vi "Obtaining Known Object Reference.vi"() -> ()   [LabVIEW 2023]
doc: "This scripting VI locates the Edit me control in the target VI and changes the Representation of the control. Because the Edit me control has a unique label, this VI can easily access it with the Open VI Object Reference function.\n\nThe Detailed Help explains how this example illustrates a general procedure for obtaining a reference in a known target VI."
uses:
  <vilib>/numeric/LVNumericRepresentation.ctl
panel:
  in  "Edit me":string="Edit me"
  # "Select Help>>Show Context Help and move the cursor over the VI icon to display help for this VI.\n\nBefore you start: Open the Detailed Help for this example to display the Obtaining References to Objects in a Known Target VI Using VI Scripting topic in the  LabVIEW Help. That topic provides additional details about how this example illustrates the general procedure for obtaining a reference to an object in a known target VI using VI Scripting.\n\nThis scripting VI locates the Edit me control in the target VI and changes the numeric representation of that control to I32. Because the Edit me control has a unique label, this VI can easily access it with the Open VI Object Reference function.\n\nOpen the target VI to observe the effects of this scripting VI. The default target VI is located in labview\\examples\\Application Control\\VI Scripting\\Finding and Modifying Objects.\n\nTo run this VI more than once, close the target VI and do not save changes."
  # "Overview: Demonstrates the use of VI Scripting to programmatically find a front panel control and change its representation.\nInstructions:\n1. Open Test - Obtain Known Object Target.vi.\n2. Run this VI.\n3. Right-click on the Edit me control on the front panel of the test VI and choose Representation. You should see that the control is now an I32 (it was previous a DBL)."
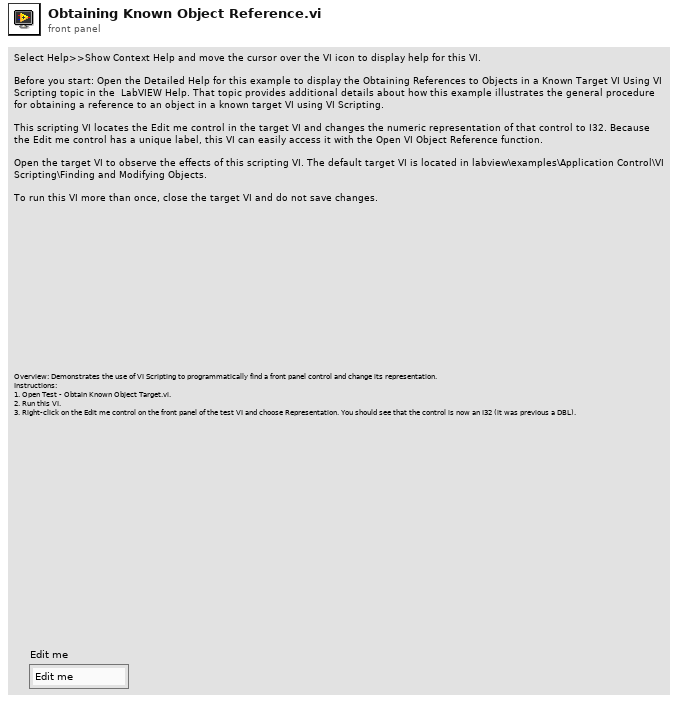
[diagram p1: front panel]
types:
  T1 = typedef "LVNumericRepresentation.ctl" = enum32{"Extended Precision", "Double Precision", "Single Precision", "Long", "Word", "Byte", "Unsigned Long", "Unsigned Word", "Unsigned Byte", "Complex Extended", "Complex Double", "Complex Single", "Quad", "Unsigned Quad", "Fixed-Point"}
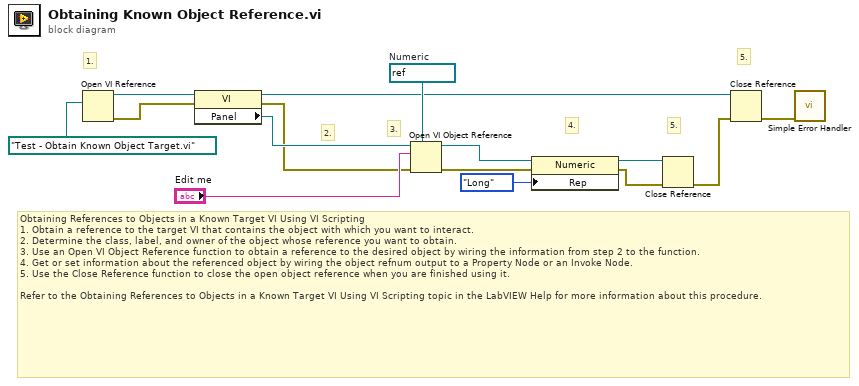
[diagram p0: block diagram]
diagram:
  w14 = refnum<vi> refnum  # Numeric
  # "5."
  # "5."
  # "4."
  # "3."
  # "2."
  # "1."
  # "Obtaining References to Objects in a Known Target VI Using VI Scripting\n1. Obtain a reference to the target VI that contains the object with which you want to interact.\n2. Determine the class, label, and owner of the object whose reference you want to obtain.\n3. Use an Open VI Object Reference function to obtain a reference to the desired object by wiring the information from step 2 to the function.\n4. Get or set information about the referenced object by wiring the object refnum output to a Property Node or an Invoke Node.\n5. Use the Close Reference function to close the open object reference when you are finished using it.\n\nRefer to the Obtaining References to Objects in a Known Target VI Using VI Scripting topic in the LabVIEW Help for more information about this procedure."
  n1 = Open VI Reference(vi path=path "Test - Obtain Known Object Target.vi") -> (vi reference=w2:refnum<vi>, error out=w3:errorcluster)  [unwired: 5 in]
  n2 = property on="Property Node" class="VI"(reference=w2, error in=w3) -> (reference out=w4:refnum<vi>, error out=w9:errorcluster, "Panel"=w11:refnum<vi>)
  n3 = Open VI Object Reference(7:w14, 8:w9, 10:"Edit me", 11:w11) -> (0:w10:errorcluster, 3:w13:refnum<vi>)
  n4 = property on="Property Node" class="Numeric"(reference=w13, error in=w10, "Rep"=LVNumericRepresentation."Long" ("new representation")) -> (reference out=w12:refnum<vi>, error out=w8:errorcluster)
  n5 = Close Reference(reference=w12, error in (no error)=w8) -> (error out=w7:errorcluster)
  n6 = Close Reference(reference=w4, error in (no error)=w7) -> (error out=w1:errorcluster)
  n7 = call <vilib>:"Simple Error Handler.vi"("error in (no error)"=w1) -> ()  [unwired: 4 in, 5 out]
